vi "PicoScope4000AWG.vi"(6 "Arbitrary Waveform Settings":T2 {"Index Mode" items=["Single", "Dual", "Quad"]}, 7 "Standard Waveform Settings":T4 {"Stop Frequency" min=0.03 max=1000000.0; "Start Frequency" min=0.03 max=1000000.0}, 8 "Unit Info":T1, 9 "General AWG Settings":T3 {"White Noise/PRBS" items=["Normal", "White Noise", "PRBS"]; "Trigger Source" items=["None", "Scope Trigger", "Aux. In", "Ext. In", "Software Trigger"]; "Trigger Type" items=["Rising", "Falling", "Gate High", "Gate Low"]; "Sweep Type" items=["Up", "Down", "Up-Down", "Down-Up"]; "Wave Type" items=["Sine", "Square", "Triangle", "Ramp Up", "Ramp Down", "Sinc", "Gaussian", "Half Sine", "DC", "White Noise", "Arbitrary"]}, 10 "Handle In":i16, 11 "error in":errorcluster) -> (0 "Trigger Source Out":u32, 1 "Arbitrary\nWaveform Graph":i16[](graph), 2 "Handle Out":i16, 3 "error out":errorcluster)   [LabVIEW 2009]
doc: "This VI can be used to control the arbitrary waveform generator. Standard waveforms can be selected or arbitrary waveform can be selected under 'Wave Type'. There are three settings clusters: general settings that apply to both arbitrary and standard waveforms, settings that apply only to standard waveforms and settings that apply only to arbitrary waveforms. It is not necessary to connect all of these clusters if only using arbitrary waveforms or only using standard waveforms are required.\n\nWhen selecting arbitrary waveform, it is necessary to specify a text file containing the wave form. This text file should have a single value on each line in the range -1 to 1. For further information on the settings, see descriptions of ps3000aSetSigGenBuiltIn and ps3000aSetSigGenArbitrary."
uses:
  ps4000.dll
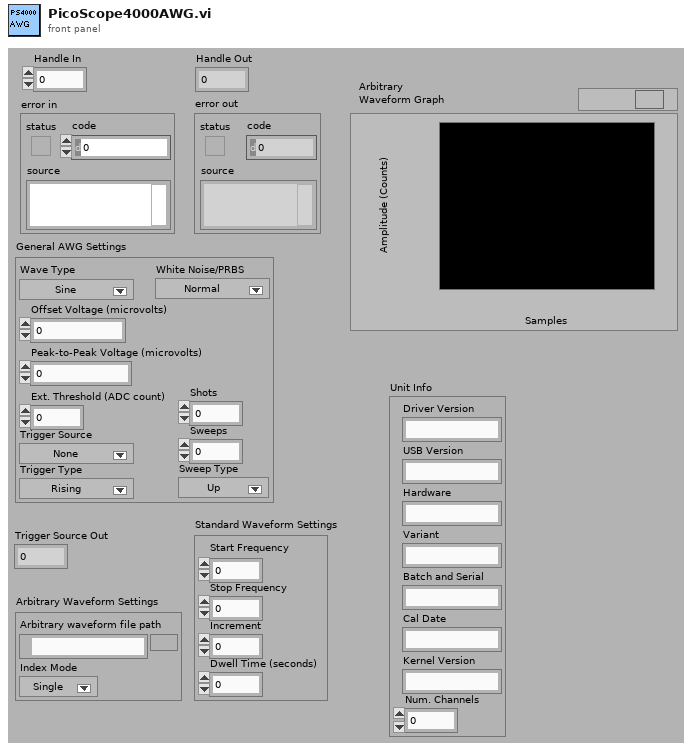
[diagram p1: front panel]
types:
  T1 = cluster{"Driver Version":string, "USB Version":string, "Hardware":string, "Variant":string, "Batch and Serial":string, "Cal Date":string, "Kernel Version":string, "Num. Channels":i16}
  T2 = cluster{"Arbirary waveform file path":path, "Index Mode":u32}
  T3 = cluster{"Peak-to-Peak Voltage (microvolts)":u32, "Offset Voltage (microvolts)":i32, "Wave Type":u32, "Sweep Type":u32, "Shots":u32, "Sweeps":u32, "Trigger Type":u32, "Trigger Source":u32, "Ext. Threshold (ADC count)":i16, "White Noise/PRBS":u32}
  T4 = cluster{"Start Frequency":dbl, "Stop Frequency":dbl, "Increment":dbl, "Dwell Time (seconds)":dbl}
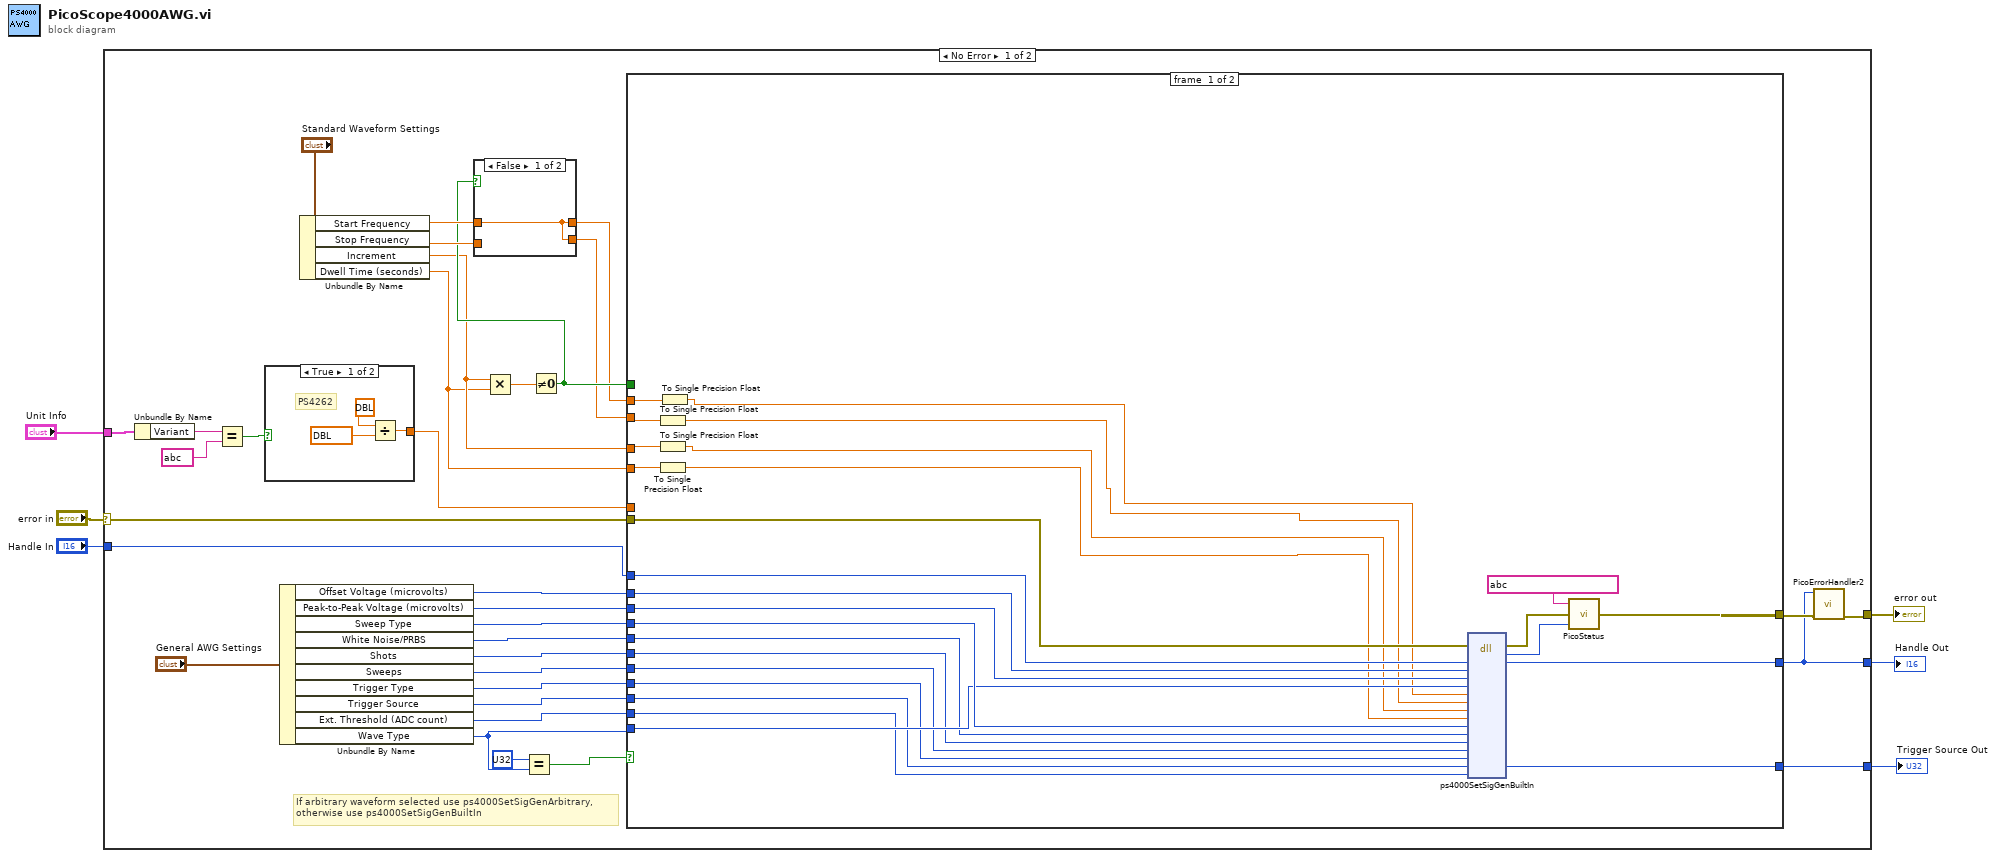
[diagram p0: block diagram]
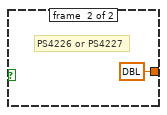
[diagram p2: hidden frame]
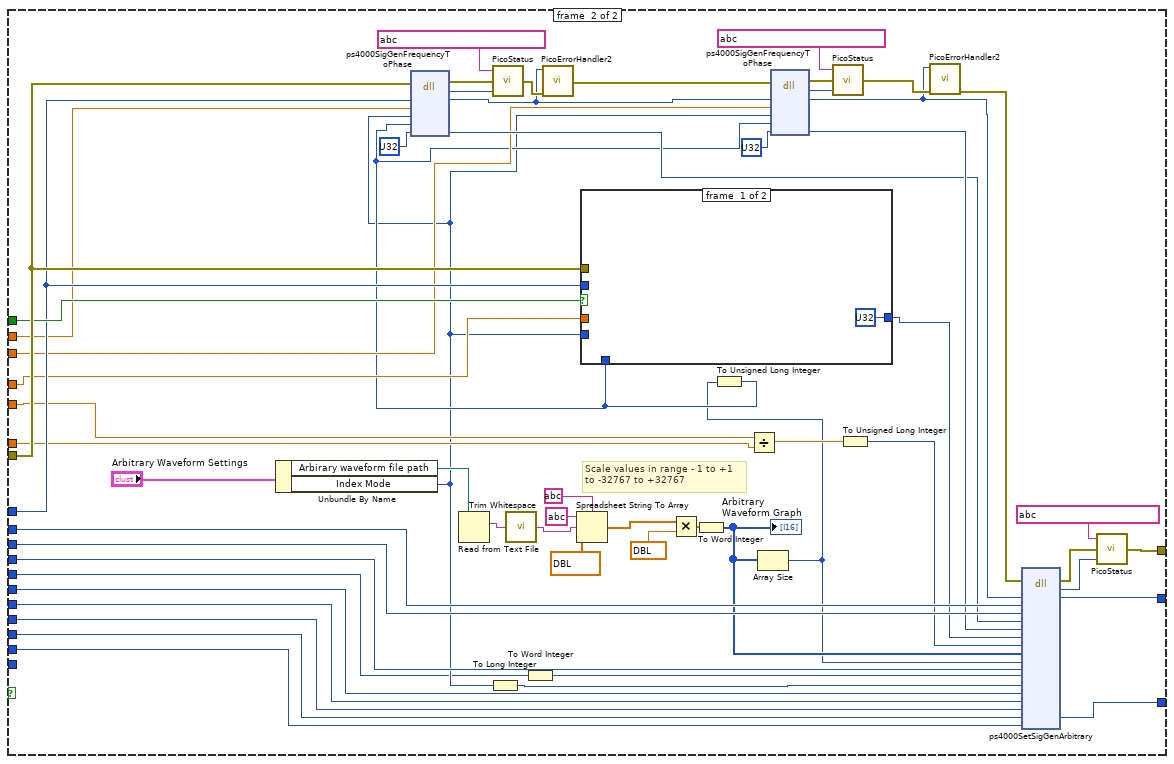
[diagram p4: hidden frame]
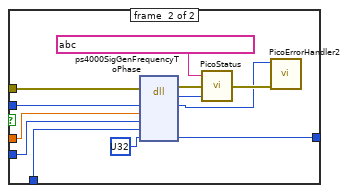
[diagram p5: hidden frame]
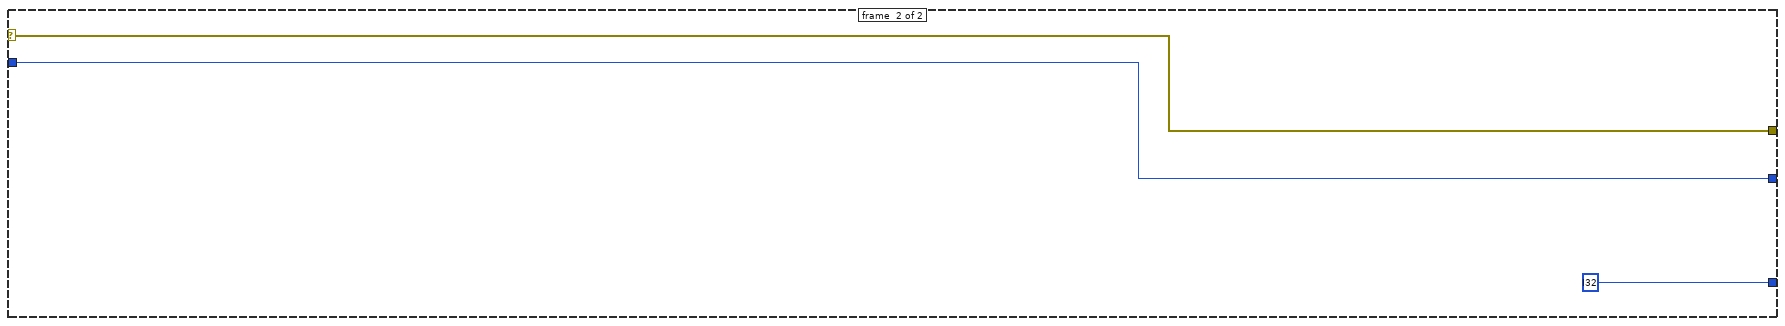
[diagram p6: hidden frame]
diagram:
  n1 = case shown="No Error" "error in" {
    selector: "error in" -> [w25 w146]
    tunnel: [w7 w145] -> w3
    tunnel: "Handle In" -> [w37 w145]
    tunnel: [w8 w146] -> w2
    tunnel: [w24 i32 ?] -> w4
    tunnel: "Unit Info" -> [w13 _]
    frame #0 {
      # "If arbitrary waveform selected use ps4000SetSigGenArbitrary, \notherwise use ps4000SetSigGenBuiltIn"
      n2 = Unbundle By Name(w13) -> ("Variant"=w12:string)
      n3 = Equal?(x=w12, y=string ?) -> (x = y?=w10:bool)
      n4 = case shown="True" w10 {
        tunnel: [w42 dbl ? ("y")] -> w14
        frame #0 {
          # "PS4262"
          n5 = Divide(x=dbl ?, y=dbl ?) -> (x/y=w42:dbl)
        }
        frame #1 {
          # "PS4226 or PS4227"
        }
      }
      n6 = Unbundle By Name("General AWG Settings") -> ("Offset Voltage (microvolts)"=w35:i32, "Peak-to-Peak Voltage (microvolts)"=w34:u32, "Sweep Type"=w33:u32, "White Noise/PRBS"=w32:u32, "Shots"=w31:u32, "Sweeps"=w30:u32, "Trigger Type"=w29:u32, "Trigger Source"=w28:u32, "Ext. Threshold (ADC count)"=w27:i16, "Wave Type"=w26:u32)
      n7 = Unbundle By Name("Standard Waveform Settings") -> ("Start Frequency"=w22:dbl, "Stop Frequency"=w21:dbl, "Increment"=w16:dbl, "Dwell Time (seconds)"=w15:dbl)
      n8 = Multiply(x=w16, y=w15) -> (x*y=w20:dbl)
      n9 = Equal?(x=u32 ?, y=w26) -> (x = y?=w39:bool)
      n10 = Not Equal To 0?(x=w20) -> (x != 0?=w19:bool)
      n11 = case shown="False" w19 {
        tunnel: [w44 w46] -> w17
        tunnel: w21 -> [_ w46]
        tunnel: w22 -> [w44 w45]
        tunnel: [w44 w45] -> w18
        frame #0 {
        }
        frame #1 {
        }
      }
      n12 = case shown="True" w39 {
        tunnel: [w72 w125] -> w7
        tunnel: w37 -> [w71 w92]
        tunnel: [w69 w122] -> w9
        tunnel: w35 -> [w67 w121]
        tunnel: w34 -> [w66 w120]
        tunnel: w33 -> [w65 w119]
        tunnel: w32 -> [w55 w79]
        tunnel: w31 -> [w63 w118]
        tunnel: w30 -> [w62 w117]
        tunnel: w29 -> [w61 w116]
        tunnel: w28 -> [w60 w115]
        tunnel: w27 -> [w59 w112]
        tunnel: w26 -> [w64 _]
        tunnel: [w58 w110] -> w24
        tunnel: w25 -> [w57 w95]
        tunnel: w19 -> [_ w93]
        tunnel: w18 -> [w54 w91]
        tunnel: w17 -> [w53 w90]
        tunnel: w16 -> [w52 w87]
        tunnel: w15 -> [w51 w88]
        tunnel: w14 -> [_ w89]
        frame #0 {
          n13 = To Single Precision Float(number=w53) -> (single precision float=w48:sgl)
          n14 = To Single Precision Float(number=w52) -> (single precision float=w49:sgl)
          n15 = To Single Precision Float(number=w51) -> (single precision float=w50:sgl)
          n16 = To Single Precision Float(number=w54) -> (single precision float=w47:sgl)
          n17 = dll-call lib="ps4000.dll" fn="ps4000SetSigGenBuiltIn" ("ps3000.dll:_ps3000_open_unit@0")(error in=w57, "handle"=w71, "offsetVoltage"=w67, "pkToPk"=w66, "waveType"=w64, "startFrequency"=w47, "stopFrequency"=w48, "increment"=w49, "dwellTime"=w50, "sweepType"=w65, "operation"=w55, "shots"=w63, "sweeps"=w62, "triggerType"=w61, "triggerSource"=w60, "extInThreshold"=w59) -> (error out=w56:errorcluster, "PICO_STATUS"=w70:u32, "handle"=w72:i16, "triggerSource"=w58:u32)  [unwired: 15 in, 1 out]
          n18 = call "PicoStatus.vi"("PICO STATUS"=w70, "error in"=w56, "source"=string ?) -> ("error out"=w69:errorcluster)
        }
        frame #1 {
          # "Scale values in range - 1 to +1 \nto -32767 to +32767"
          n19 = Unbundle By Name("Arbitrary Waveform Settings") -> ("Arbirary waveform file path"=w113:path, "Index Mode"=w80:u32)
          n20 = Read from Text File(file (use dialog)=w113) -> (text=w82:string)  [unwired: 3 in, 3 out]
          n21 = To Long Integer(number=w80) -> (32bit integer=w78:i32)
          n22 = call <vilib>:"Trim Whitespace.vi"("string"=w82) -> ("trimmed string"=w81:string)  [unwired: 1 in]
          n23 = To Word Integer(number=w79) -> (16bit integer=w77:i16)
          n24 = Spreadsheet String To Array(delimiter (Tab)=string ?, format string=string ?, spreadsheet string=w81, array type (2D Dbl)=dbl[] ?) -> (array=w126:dbl[])
          n25 = Multiply(x=w126, y=dbl ? ("deltaPhaseIncrement")) -> (x*y=w108:dbl[])
          n26 = To Word Integer(number=w108) -> (16bit integer=w111:i16[])
          "Arbitrary\nWaveform Graph" <- w111
          n27 = Divide(x=w88, y=w89) -> (x/y=w86:dbl)
          n28 = Array Size(array=w111) -> (size(s)=w83:i32)
          n29 = To Unsigned Long Integer(number=w83) -> (unsigned 32bit integer=w84:u32)
          n30 = dll-call lib="ps4000.dll" fn="ps4000SigGenFrequencyToPhase" ("ps3000.dll:_ps3000_open_unit@0")(error in=w95, "handle"=w92, "frequency"=w91, "indexMode"=w80, "bufferLength"=w84, "phase"=u32 ?) -> (error out=w105:errorcluster, "PICO_STATUS"=w104:u32, "handle"=w76:i16, "phase"=w94:u32)  [unwired: 5 in, 1 out]
          n31 = call "PicoStatus.vi"("PICO STATUS"=w104, "error in"=w105, "source"=string ?) -> ("error out"=w107:errorcluster)
          n32 = call "PicoErrorHandler2.vi"("error in (no error)"=w107, "handle In"=w76) -> ("error out"=w100:errorcluster)  [unwired: 9 in]
          n33 = case shown="True" w93 {
            tunnel: w95 -> [_ w140]
            tunnel: w92 -> [_ w139]
            tunnel: w87 -> [_ w138]
            tunnel: w84 -> [_ w136]
            tunnel: [u32 ? ("phase") w135] -> w96
            tunnel: w80 -> [_ w134]
            frame #0 {
            }
            frame #1 {
              n34 = dll-call lib="ps4000.dll" fn="ps4000SigGenFrequencyToPhase" ("ps3000.dll:_ps3000_open_unit@0")(error in=w140, "handle"=w139, "frequency"=w138, "indexMode"=w134, "bufferLength"=w136, "phase"=u32 ?) -> (error out=w142:errorcluster, "PICO_STATUS"=w143:u32, "handle"=w132:i16, "phase"=w135:u32)  [unwired: 5 in, 1 out]
              n35 = call "PicoStatus.vi"("PICO STATUS"=w143, "error in"=w142, "source"=string ?) -> ("error out"=w133:errorcluster)
              n36 = call "PicoErrorHandler2.vi"("error in (no error)"=w133, "handle In"=w132) -> ()  [unwired: 9 in, 1 out]
            }
          }
          n37 = dll-call lib="ps4000.dll" fn="ps4000SigGenFrequencyToPhase" ("ps3000.dll:_ps3000_open_unit@0")(error in=w100, "handle"=w76, "frequency"=w90, "indexMode"=w80, "bufferLength"=w84, "phase"=u32 ?) -> (error out=w102:errorcluster, "PICO_STATUS"=w101:u32, "handle"=w74:i16, "phase"=w97:u32)  [unwired: 5 in, 1 out]
          n38 = call "PicoStatus.vi"("PICO STATUS"=w101, "error in"=w102, "source"=string ?) -> ("error out"=w75:errorcluster)
          n39 = To Unsigned Long Integer(number=w86) -> (unsigned 32bit integer=w85:u32)
          n40 = call "PicoErrorHandler2.vi"("error in (no error)"=w75, "handle In"=w74) -> ("error out"=w73:errorcluster)  [unwired: 9 in]
          n41 = dll-call lib="ps4000.dll" fn="ps4000SetSigGenArbitrary" ("ps3000.dll:_ps3000_open_unit@0")(error in=w73, "handle"=w74, "offsetVoltage"=w121, "pkToPk"=w120, "startDeltaPhase"=w94, "stopDeltaPhase"=w97, "deltaPhaseIncrement"=w96, "dwellCount"=w85, "arbitraryWaveform"=w111, "arbitraryWaveformSize"=w83, "sweepType"=w119, "operation"=w77, "indexMode"=w78, "shots"=w118, "sweeps"=w117, "triggerType"=w116, "triggerSource"=w115, "extInThreshold"=w112) -> (error out=w109:errorcluster, "PICO_STATUS"=w124:u32, "handle"=w125:i16, "triggerSource"=w110:u32)  [unwired: 17 in, 1 out]
          n42 = call "PicoStatus.vi"("PICO STATUS"=w124, "error in"=w109, "source"=string ?) -> ("error out"=w122:errorcluster)
        }
      }
      n43 = call "PicoErrorHandler2.vi"("error in (no error)"=w9, "handle In"=w7) -> ("error out"=w8:errorcluster)  [unwired: 9 in]
    }
    frame #1 {
    }
  }
  "Handle Out" <- w3
  "error out" <- w2
  "Trigger Source Out" <- w4
